vi "R&S Set RF.vi"(4 "amplitude (mV)":i32, 5 "error in (no error)":errorcluster, 6 "modulation (kHz)":i32, 7 "center frequency (MHz)":dbl, 8 "address":string) -> (0 "error out":errorcluster, 3 "address out":string)   [LabVIEW 2019]
doc: "This device configures the Rohde & Schwarz RF Generator for use. The central frequency, modulation, RF power, and GPIB address are taken from the QCA Global."
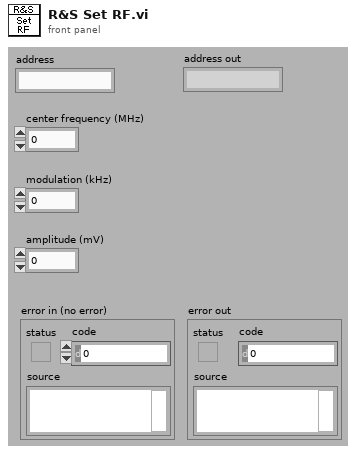
[diagram p1: front panel]
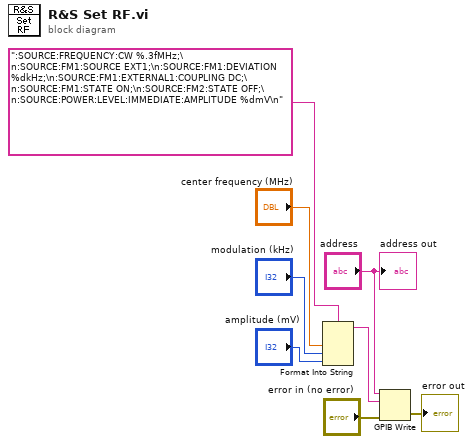
[diagram p0: block diagram]
diagram:
  n1 = Format Into String(format string=":SOURCE:FREQUENCY:CW %.3fMHz;\n:SOURCE:FM1:SOURCE EXT1;\n:SOURCE:FM1:DEVIATION %dkHz;\n:SOURCE:FM1:EXTERNAL1:COUPLING DC;\n:SOURCE:FM1:STATE ON;\n:SOURCE:FM2:STATE OFF;\n:SOURCE:POWER:LEVEL:IMMEDIATE:AMPLITUDE %dmV\n", "center frequency (MHz)", "modulation (kHz)", "amplitude (mV)") -> (resulting string=w7:string)  [unwired: 2 in, 1 out]
  n2 = GPIB Write(0:"address", 1:w7, 3:"error in (no error)") -> (6:→"error out":errorcluster)  [unwired: 2 in, 1 out]
  "address out" <- "address"
